vi "TestEnsureIgorStringFormat.vi"(8 "error in (no error)":errorcluster) -> (0 "error out":errorcluster)   [LabVIEW 2019]
uses:
  <vilib>/addons/_JKI Toolkits/Caraya/classes/Assert/Assert Equal Value and Type_Variant.vi
  <vilib>/addons/_JKI Toolkits/Caraya/classes/Test/Test.lvclass
  <vilib>/addons/_JKI Toolkits/Caraya/classes/Assert/Assert.lvclass
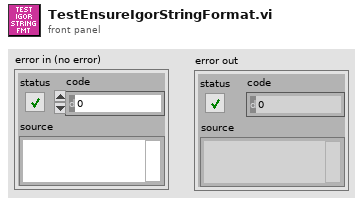
[diagram p1: front panel]
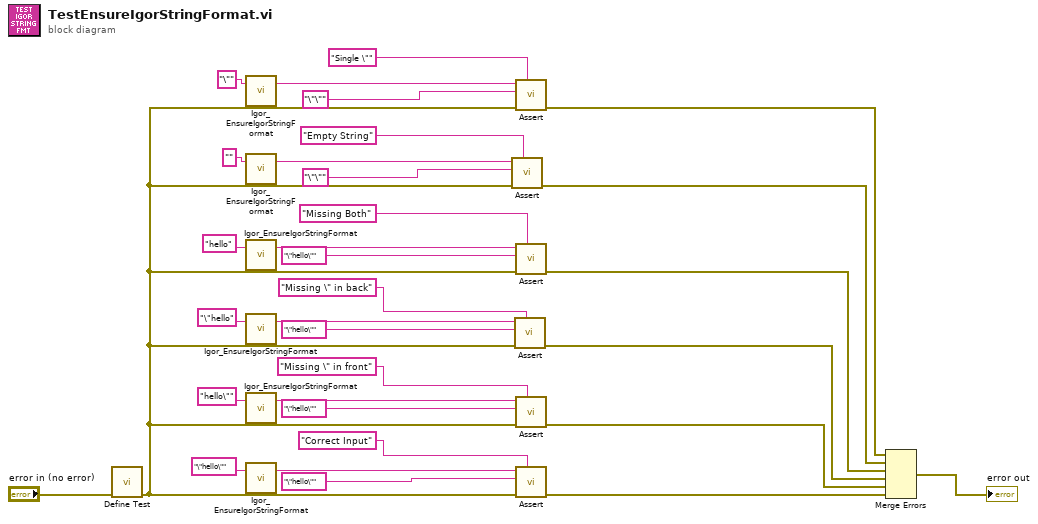
[diagram p0: block diagram]
diagram:
  n1 = call <vilib>:"Define Test.vi"("error in (no error)"="error in (no error)") -> ("error out"=w25:errorcluster)  [unwired: 9 in, 1 out]
  n2 = call "Igor_EnsureIgorStringFormat.vi"("Value"="\"") -> ("Value"=w12:string)  [unwired: 2 in]
  n3 = call "Igor_EnsureIgorStringFormat.vi"("Value"="") -> ("Value"=w10:string)  [unwired: 2 in]
  n4 = call "Igor_EnsureIgorStringFormat.vi"("Value"="hello") -> ("Value"=w8:string)  [unwired: 2 in]
  n5 = call "Igor_EnsureIgorStringFormat.vi"("Value"="\"hello") -> ("Value"=w6:string)  [unwired: 2 in]
  n6 = call "Igor_EnsureIgorStringFormat.vi"("Value"="hello\"") -> ("Value"=w4:string)  [unwired: 2 in]
  n7 = call "Igor_EnsureIgorStringFormat.vi"("Value"="\"hello\"") -> ("Value"=w2:string)  [unwired: 2 in]
  n8 = call-poly <vilib>:"Assert.vi"("Label"="Empty String", "error in (no error)"=w25, "Y"="\"\"" ("Label"), "X"=w10) -> ("error out"=w20:errorcluster)  [unwired: 6 in, 1 out]
  n9 = call-poly <vilib>:"Assert.vi"("Label"="Missing \" in back", "error in (no error)"=w25, "Y"="\"hello\"" ("Value"), "X"=w6) -> ("error out"=w22:errorcluster)  [unwired: 6 in, 1 out]
  n10 = call-poly <vilib>:"Assert.vi"("Label"="Single \"", "error in (no error)"=w25, "Y"="\"\"" ("Label"), "X"=w12) -> ("error out"=w19:errorcluster)  [unwired: 6 in, 1 out]
  n11 = call-poly <vilib>:"Assert.vi"("Label"="Missing Both", "error in (no error)"=w25, "Y"="\"hello\"" ("Value"), "X"=w8) -> ("error out"=w21:errorcluster)  [unwired: 6 in, 1 out]
  n12 = call-poly <vilib>:"Assert.vi"("Label"="Missing \" in front", "error in (no error)"=w25, "Y"="\"hello\"" ("Value"), "X"=w4) -> ("error out"=w23:errorcluster)  [unwired: 6 in, 1 out]
  n13 = call-poly <vilib>:"Assert.vi"("Label"="Correct Input", "error in (no error)"=w25, "Y"="\"hello\"" ("Value"), "X"=w2) -> ("error out"=w24:errorcluster)  [unwired: 6 in, 1 out]
  n14 = Merge Errors(w19, w20, w21, w22, w23, w24) -> (→"error out":errorcluster)
